vi "VISA_INITIALIZE.vi"(4 "IDN? (T)":bool=TRUE, 8 "error in":errorcluster {"code" format="%.0x"}, 11 "Session In":refnum<visa-resource-name>="GPIB0::10::INSTR") -> (0 "error out":errorcluster {"code" format="%.0x"}, 1 "SN":string, 2 "Model":string, 3 "Session Out":refnum<visa-resource-name>, 5 "STB":string, 7 "Mfr":string)   [LabVIEW 2018]
doc: "This sub vi Initializes the VISA Instrument and optionally queries for idn"
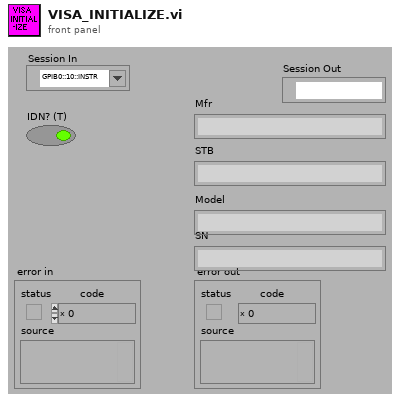
[diagram p1: front panel]
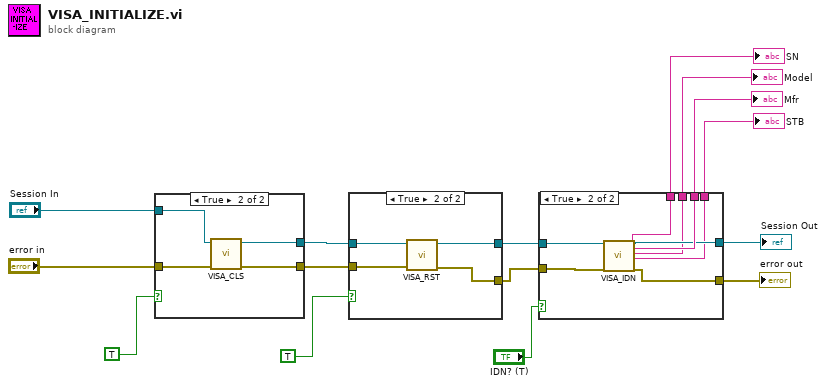
[diagram p0: block diagram]
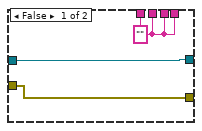
[diagram p2: hidden frame]
diagram:
  n1 = case shown="True" TRUE {
    tunnel: [w17 w21] -> w15
    tunnel: [w16 w20] -> w14
    tunnel: "error in" -> [w16 w19]
    tunnel: "Session In" -> [w17 w18]
    frame False {
    }
    frame True {
      n2 = call "VISA_CLS.vi"("error in"=w19, "Session In"=w18) -> ("error out"=w20:errorcluster, "Session Out"=w21:refnum<visa-resource-name>)  [unwired: 8 in]
    }
  }
  n3 = case shown="True" TRUE {
    tunnel: w15 -> [w22 w27]
    tunnel: w14 -> [w23 w26]
    tunnel: [w23 w25] -> w8
    tunnel: [w22 w24] -> w11
    frame False {
    }
    frame True {
      n4 = call "VISA_RST.vi"("error in"=w26, "Session In"=w27) -> ("error out"=w25:errorcluster, "Session Out"=w24:refnum<visa-resource-name>)  [unwired: 8 in]
    }
  }
  n5 = case shown="True" "IDN? (T)" {
    tunnel: [w28 w38] -> w13
    tunnel: [w28 w32] -> w12
    tunnel: w11 -> [w30 w37]
    tunnel: [w30 w36] -> w10
    tunnel: [w29 w35] -> w9
    tunnel: w8 -> [w29 w34]
    tunnel: [w28 w33] -> w5
    tunnel: [w28 w31] -> w4
    frame False {
      w28 = "" ("SN")
    }
    frame True {
      n6 = call "VISA_IDN.vi"("Session In"=w37, "error in"=w34) -> ("Session Out"=w36:refnum<visa-resource-name>, "Mfr"=w38:string, "Model"=w32:string, "Ver"=w31:string, "SN"=w33:string, "error out"=w35:errorcluster)  [unwired: 11 in, 1 out]
    }
  }
  "error out" <- w9
  "Session Out" <- w10
  "STB" <- w4
  "SN" <- w5
  "Mfr" <- w13
  "Model" <- w12
